vi "Get Session from ClientID.vi"(8 "error in (no error)":errorcluster, 10 "Client ID":string, 11 "MQTT_Base in":refnum<class "MQTT_Base.lvclass">) -> (0 "error out":errorcluster, 1 "found?":bool, 2 "SessionMailbox":refnum<queue>, 3 "MQTT_Base out":refnum<class "MQTT_Base.lvclass">)   [LabVIEW 2013, in "MQTT Server.lvlib" / "MQTT_Base.lvclass"]
uses:
  MQTT_Base.lvclass
  Response -- cluster.ctl
  Control Packets/ControlPacket/ControlPacket.lvclass
  MQTT_Base.lvclass/MQTT_Base.ctl
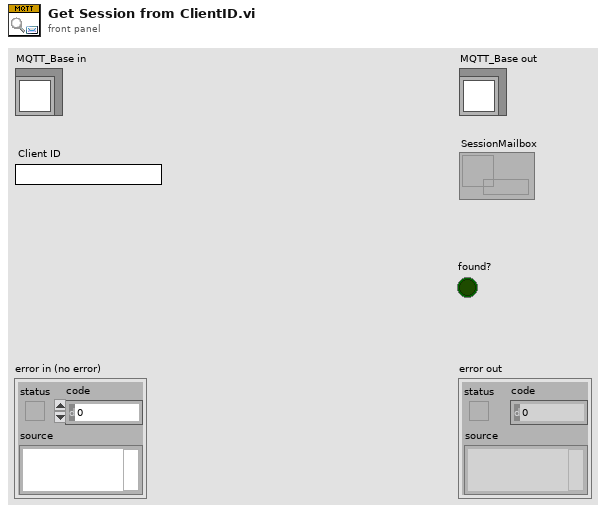
[diagram p1: front panel]
types:
  T1 = typedef "MQTT Server.lvlib/MQTT_Base.lvclass/SessionRef -- cluster.ctl" = cluster{"ClientID":string, "SessionMailbox":refnum<queue>}
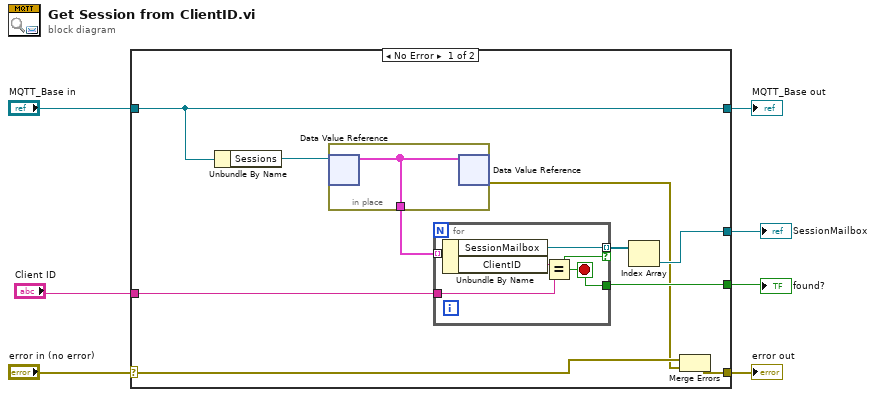
[diagram p0: block diagram]
diagram:
  n1 = case shown="No Error" "error in (no error)" {
    selector: "error in (no error)" -> [w10 w25]
    tunnel: [w8 w25] -> w6
    tunnel: [w17 w24] -> w4
    tunnel: "MQTT_Base in" -> [w17 w24]
    tunnel: "Client ID" -> [w14 _]
    tunnel: [w11 _] -> w2
    tunnel: [w12 _] -> w1
    frame No Error {
      n2 = Unbundle By Name(w17) -> ("Sessions"=w16:refnum<data-value>)
      n3 = in-place {
        in-place-border: [w23] -> w15
        n4 = in-place-dvr #1(w16) -> (w23:T1[])  [unwired: 1 out]
        n5 = in-place-dvr #1(w23) -> (w9:errorcluster)  [unwired: 1 out]
      }
      n6 = for {
        tunnel: w15 -> [w22] mode=indexing
        tunnel: w14 -> [w20]
        tunnel: [w19] -> w13 mode=indexing if=w18
        tunnel: [w18] -> w11
        stop <- w18 stop-if-true
        n7 = Unbundle By Name(w22) -> ("SessionMailbox"=w19:refnum<queue>, "ClientID"=w21:string)
        n8 = Equal?(x=w21, y=w20) -> (x = y?=w18:bool)
      }
      n9 = Index Array(array=w13) -> (element=w12:refnum<queue>)  [unwired: 1 in]
      n10 = Merge Errors(w10, w9) -> (w8:errorcluster)
    }
    frame Error {
    }
  }
  "error out" <- w6
  "MQTT_Base out" <- w4
  "SessionMailbox" <- w1
  "found?" <- w2
